vi "stop.vi"(3 "error in (no error)":errorcluster, 4 "stop":bool, 5 "niDAQmxAO in":refnum<class "niDAQmxAO.lvclass">) -> (0 "error out":errorcluster, 1 "Stopped":bool, 2 "niDAQmxAO out":refnum<class "niDAQmxAO.lvclass">)   [LabVIEW 2009, in "Hardware.lvlib" / "Channels.lvlib" / "niDAQmxAO.lvclass"]
uses:
  niDAQmxAO.lvclass
  niDAQmxAO.lvclass/niDAQmxAO.ctl
  C:/Program Files/National Instruments/LabVIEW 2009/resource/objmgr/daqmx.rc
panel:
  out "SampQuant.SampPerChan":dbl
  out "TotalSampPerChanGenerated":dbl
  out "for testing only":bool=TRUE
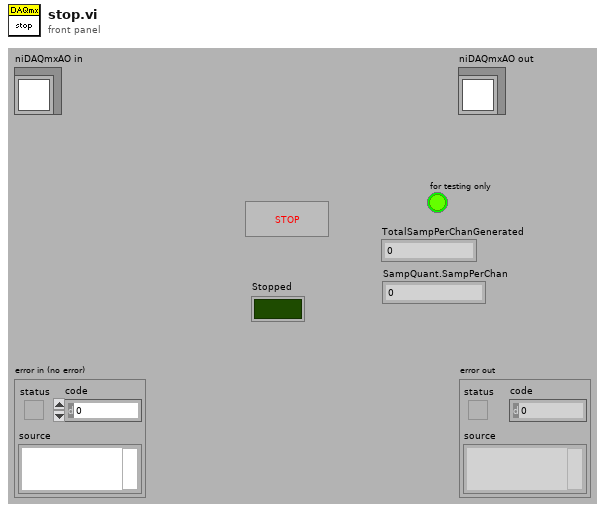
[diagram p1: front panel]
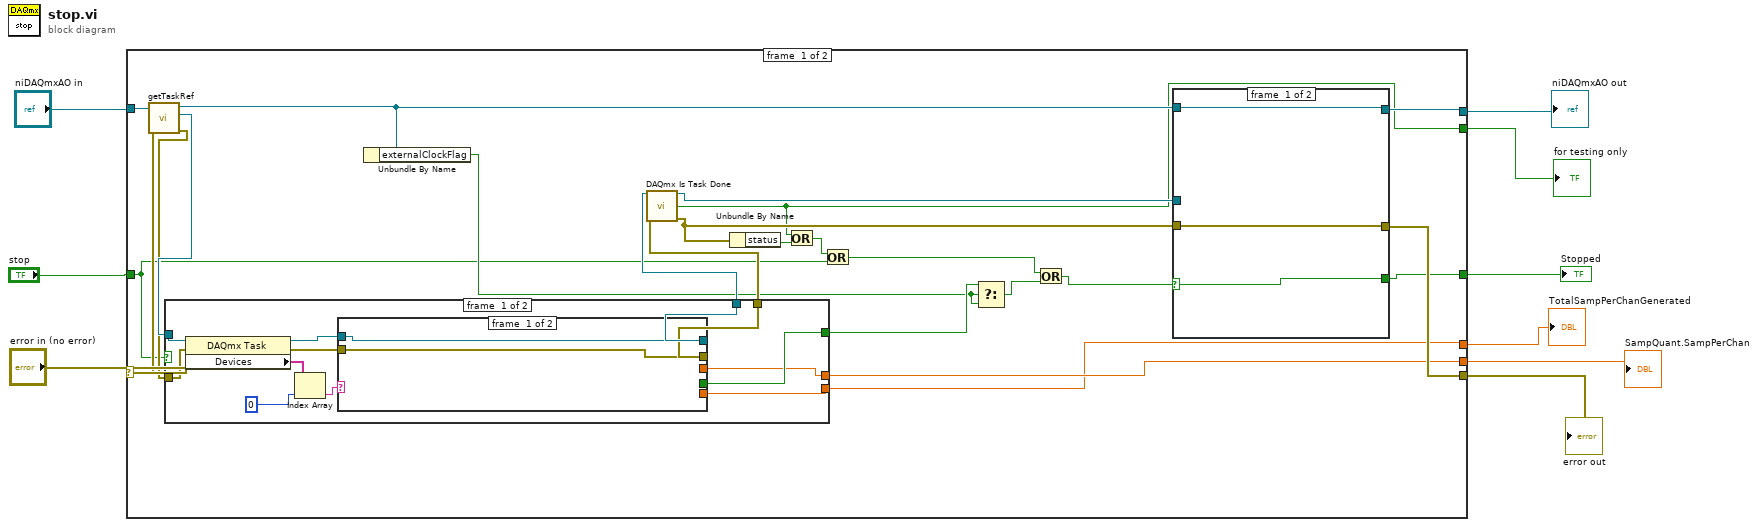
[diagram p0: block diagram]
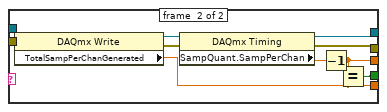
[diagram p2: hidden frame]
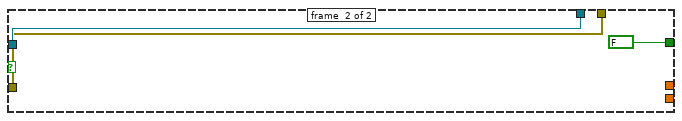
[diagram p3: hidden frame]
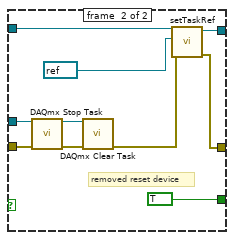
[diagram p4: hidden frame]
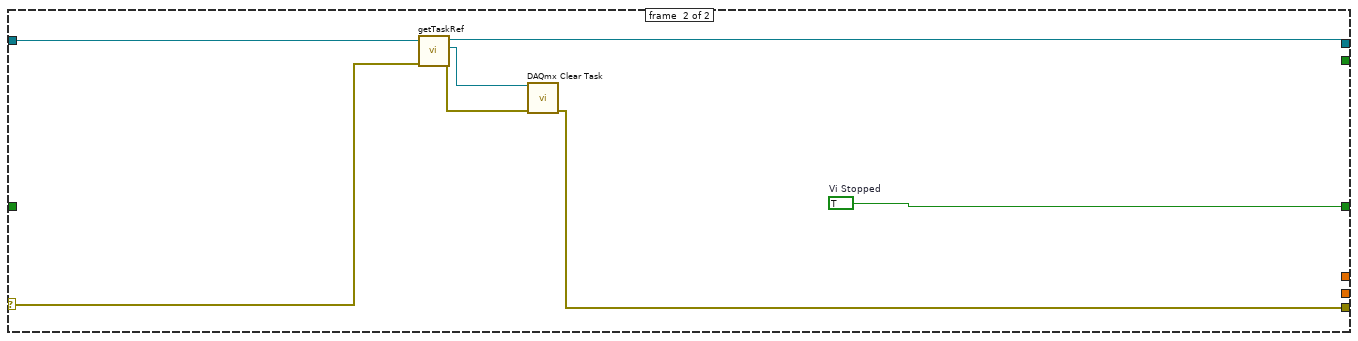
[diagram p5: hidden frame]
diagram:
  n1 = case shown="No Error" "error in (no error)" {
    selector: "error in (no error)" -> [w31 w78]
    tunnel: [w28 w74] -> w8
    tunnel: [w12 w75] -> w6
    tunnel: "niDAQmxAO in" -> [w32 w79]
    tunnel: "stop" -> [w14 _]
    tunnel: [w25 w73] -> w4
    tunnel: [w11 _] -> w3
    tunnel: [w19 _] -> w2
    tunnel: [w20 _] -> w1
    frame #0 {
      n2 = call "getTaskRef.vi"("error in (no error)"=w31, "niDAQmxAO.lvclass in"=w32) -> ("error out"=w23:errorcluster, "DAQmx Task Ref"=w24:refnum<k21>, "niDAQmxAO.lvclass out"=w13:refnum<class "niDAQmxAO.lvclass">)  [unwired: 7 in]
      n3 = case shown="False" w14 {
        tunnel: w24 -> [w41 w59]
        tunnel: w23 -> [w40 w58]
        tunnel: [w44 w59] -> w22
        tunnel: [w43 w58] -> w21
        tunnel: [w33 _] -> w20
        tunnel: [w42 _] -> w19
        tunnel: [w34 FALSE] -> w16
        frame #0 {
          n4 = property class="DAQmx Task"(reference=w41, error in=w40) -> (reference out=w39:refnum<k21>, error out=w38:errorcluster, "Devices"=w36:tag[])
          n5 = Index Array(array=w36, index=0) -> (element=w35:tag)
          n6 = case shown="\"Ao32\", \"Ao8\", \"DAQ\"" w35 {
            tunnel: [w46 w55] -> w44
            tunnel: [w45 w53] -> w43
            tunnel: [_ w49] -> w42
            tunnel: w39 -> [w46 w52]
            tunnel: w38 -> [w45 w51]
            tunnel: [_ w48] -> w34
            tunnel: [_ w47] -> w33
            frame #0 {
            }
            frame #1 {
              n7 = property class="DAQmx Write"(reference=w52, error in=w51) -> (reference out=w56:refnum<k21>, error out=w54:errorcluster, "TotalSampPerChanGenerated"=w49:dbl)
              n8 = property class="DAQmx Timing"(reference=w56, error in=w54) -> (reference out=w55:refnum<k21>, error out=w53:errorcluster, "SampQuant.SampPerChan"=w50:dbl)
              n9 = Decrement(x=w50) -> (x-1=w47:dbl)
              n10 = Equal?(x=w47, y=w49) -> (x = y?=w48:bool)
            }
          }
        }
        frame #1 {
        }
      }
      n11 = Unbundle By Name(w13) -> ("externalClockFlag"=w15:bool)
      n12 = call <vilib>:"DAQmx Is Task Done.vi"("task/channels in"=w22, "error in"=w21) -> ("task out"=w30:refnum<k21>, "task done?"=w11:bool, "error out"=w29:errorcluster)  [unwired: 11 in]
      n13 = Unbundle By Name(w29) -> ("status"=w26:bool)
      n14 = Or(x=w11, y=w26) -> (x .or. y?=w27:bool)
      n15 = Or(x=w27, y=w14) -> (x .or. y?=w17:bool)
      n16 = Select(t=w16, s=w15, f=w15) -> (s? t:f=w18:bool)
      n17 = Or(x=w17, y=w18) -> (x .or. y?=w10:bool)
      n18 = case shown="True" w10 {
        selector: w10 -> [w61 _]
        tunnel: w30 -> [_ w68]
        tunnel: w29 -> [w62 w71]
        tunnel: [w62 w64] -> w28
        tunnel: [w61 TRUE] -> w25
        tunnel: w13 -> [w60 w67]
        tunnel: [w60 w63] -> w12
        frame #0 {
        }
        frame #1 {
          # "removed reset device"
          n19 = call <vilib>:"DAQmx Stop Task.vi"("task/channels in"=w68, "error in"=w71) -> ("task out"=w69:refnum<k21>, "error out"=w70:errorcluster)  [unwired: 12 in]
          n20 = call <vilib>:"DAQmx Clear Task.vi"("task in"=w69, "error in"=w70) -> ("error out"=w65:errorcluster)  [unwired: 13 in]
          n21 = call "setTaskRef.vi"("error in (no error)"=w65, "DAQmx Task Ref"=refnum<k21> refnum ("task out"), "niDAQmxAO.lvclass in"=w67) -> ("error out"=w64:errorcluster, "niDAQmxAO.lvclass out"=w63:refnum<class "niDAQmxAO.lvclass">)  [unwired: 7 in]
        }
      }
    }
    frame #1 {
      w73 = TRUE  # Vi Stopped
      n22 = call "getTaskRef.vi"("error in (no error)"=w78, "niDAQmxAO.lvclass in"=w79) -> ("error out"=w76:errorcluster, "DAQmx Task Ref"=w77:refnum<k21>, "niDAQmxAO.lvclass out"=w75:refnum<class "niDAQmxAO.lvclass">)  [unwired: 7 in]
      n23 = call <vilib>:"DAQmx Clear Task.vi"("task in"=w77, "error in"=w76) -> ("error out"=w74:errorcluster)  [unwired: 13 in]
    }
  }
  "error out" <- w8
  "niDAQmxAO out" <- w6
  "Stopped" <- w4
  "for testing only" <- w3
  "TotalSampPerChanGenerated" <- w2
  "SampQuant.SampPerChan" <- w1
